vi "Param redefine.vi"(6 "conninfo":T2={"host"="localhost", "port"="5432", "client_encoding"="WIN1251", "dbname"="data", "user"="postgres", "password"=""}, 8 "error in (no error)":errorcluster, 9 "ParamTable":string="par_3", 10 "Parameters":string[](array[string]), 11 "Param in":T1) -> (0 "error":errorcluster, 3 "Param out":T1)   [LabVIEW 2019, in "Inputs.lvlib"]
uses:
  Inputs.lvlib
  Ctl/Param.ctl
  Database/ctl/Coninfo.ctl
  Ctl/ParamColumns.ctl
  Database/select_initial.vi
  Database/PostgreSQL2LabVIEW/libpqUtility/src/PQclose.vi
  Database/PostgreSQL2LabVIEW/libpqUtility/src/PQconnect.vi
  Database/PostgreSQL2LabVIEW/libpqlv/src/PQfinish.vi
  Database/PostgreSQL2LabVIEW/libpqlv/src/PQconnectdb.vi
  Database/PostgreSQL2LabVIEW/libpqlv/src/PQerrorMessage.vi
  Database/PostgreSQL2LabVIEW/libpqlv/src/PQstatus.vi
  <vilib>/dlg_ctls.llb/Space Constant.vi
  Database/PostgreSQL2LabVIEW/libpqUtility/src/PQgetTable.vi
  Database/Progress.vi
  Database/PostgreSQL.lvlib
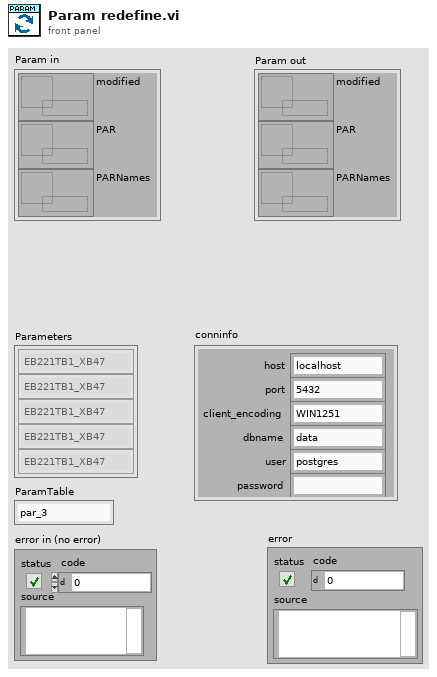
[diagram p1: front panel]
types:
  T1 = typedef "Inputs.lvlib/Param.ctl" = cluster{"modified":refnum<data-value>, "PAR":refnum<data-value>, "PARNames":refnum<data-value>}
  T2 = typedef "PostgreSQL.lvlib/Coninfo.ctl" = cluster{"host":string, "port":string, "client_encoding":string, "dbname":string, "user":string, "password":string}
  T3 = typedef "Inputs.lvlib/ParamColumns.ctl" = enum16{"value", "value_range_min", "value_range_max", "d", "fname", "value_units", "fcode", "fcodef", "fcode_full"}
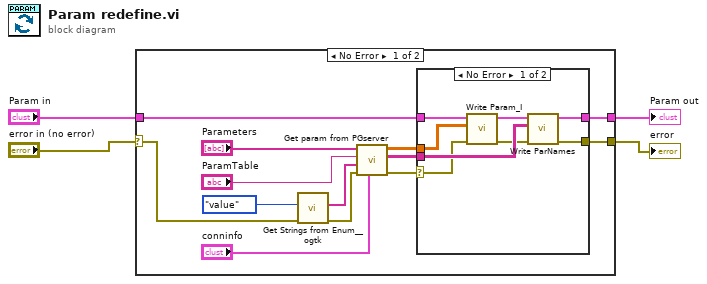
[diagram p0: block diagram]
diagram:
  n1 = case shown="No Error" "error in (no error)" {
    selector: "error in (no error)" -> [w7 w29]
    tunnel: [w12 w29] -> w4
    tunnel: "Param in" -> [w10 w28]
    tunnel: [w9 w28] -> w3
    frame No Error {
      n2 = call <userlib>:"Get Strings from Enum__ogtk.vi"("error in (no error)"=w7, "Enum"=ParamColumns."value" ("ParamColumns")) -> ("error out"=w6:errorcluster, "Enum Strings"=w5:string[])  [unwired: 6 in, 2 out]
      n3 = call "Get param from PGserver.vi"("conninfo"="conninfo", "error in (no error)"=w6, "ParamColumns"=w5, "ParamTable"="ParamTable", "Parameters"="Parameters") -> ("error out"=w14:errorcluster, "Names table"=w15:string[][], "Parameters table"=w16:dbl[][])  [unwired: 4 in]
      n4 = case shown="No Error" w14 {
        selector: w14 -> [w20 w26]
        tunnel: w16 -> [w22 _]
        tunnel: w15 -> [w25 _]
        tunnel: [w19 w26] -> w12
        tunnel: w10 -> [w24 w27]
        tunnel: [w18 w27] -> w9
        frame No Error {
          n5 = call "Write Param_I.vi"("error in (no error)"=w20, "Param"=w22, "Param in"=w24) -> ("error out"=w21:errorcluster, "Param out"=w23:T1)  [unwired: 7 in]
          n6 = call "Write ParNames.vi"("error in (no error)"=w21, "PARNames"=w25, "Param in"=w23) -> ("error out"=w19:errorcluster, "Param out"=w18:T1)  [unwired: 7 in]
        }
        frame Error {
        }
      }
    }
    frame Error {
    }
  }
  "Param out" <- w3
  "error" <- w4
